vi "get_multiramp_soak_profile_configuration.vi"(8 "error in (no error)":errorcluster, 9 "Segment number":u8 max=15, 10 "Program number":u8 max=99, 11 "connection ID":refnum<k5>) -> (0 "error out":errorcluster, 2 "Tracking enabled":bool, 3 "connection ID out":refnum<k5>)   [LabVIEW 2018]
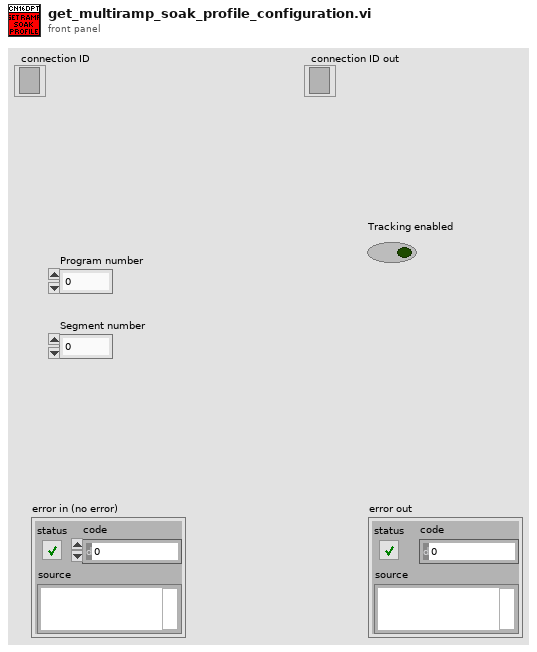
[diagram p1: front panel]
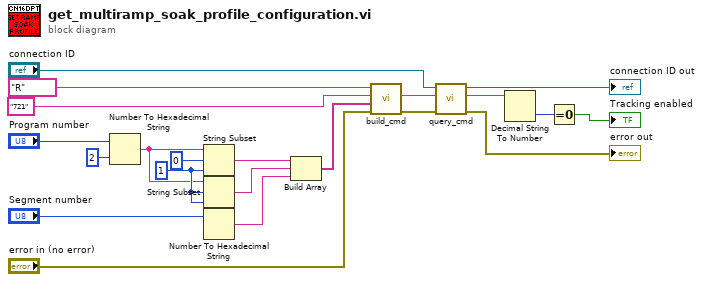
[diagram p0: block diagram]
diagram:
  w10 = 1 ("length (rest)")
  n1 = Number To Hexadecimal String(1:i16 2 ("width (-)"), 2:"Program number") -> (0:w9:string)
  n2 = String Subset(string=w9, offset (0)=0, length (rest)=w10) -> (substring=w8:string)
  n3 = String Subset(string=w9, offset (0)=w10, length (rest)=w10) -> (substring=w7:string)
  n4 = Number To Hexadecimal String(2:"Segment number") -> (0:w6:string)  [unwired: 1 in]
  n5 = Build Array(w8, w7, w6) -> (w15:string[])
  n6 = call "build_cmd.vi"("error in (no error)"="error in (no error)", "Parameter list"=w15, "Command ID"="721", "Command class"="R") -> ("error out"=w18:errorcluster, "Command"=w17:string)  [unwired: 6 in]
  n7 = call "query_cmd.vi"("error in (no error)"=w18, "Command"=w17, "connection ID"="connection ID") -> ("error out"=→"error out":errorcluster, "Response"=w5:string, "connection ID out"=→"connection ID out":refnum<k5>)  [unwired: 6 in]
  n8 = Decimal String To Number(string=w5) -> (number=w4:i32)  [unwired: 2 in, 1 out]
  n9 = Equal To 0?(x=w4) -> (x = 0?=→"Tracking enabled":bool)
